vi "LTVDiffDriveCtrl_Pack_Ctrl_Params.vi"(4 "Max right vel ctrl effort V":dbl=12.0, 6 "Max left vel ctrl effort V":dbl=12.0, 7 "Desired X Pos Ctrl Tol M":dbl=0.0625, 8 "Desired Right Vel Ctrl Tol M/S":dbl=0.3, 9 "Desired Left Vel Ctrl Tol M/S":dbl=0.3, 10 "Desired Heading Ctrl Tol Rad":dbl=0.2, 11 "Desired Y Pos Meas Tol M":dbl=0.125) -> (3 "LTV_DiffDriveCtrl_Control":T1={"Max left vel ctrl effort V"=0.0, "Desired Heading Ctrl Tol Rad"=0.0, "Desired Y Pos Meas Tol M"=0.0, "Desired X Pos Ctrl Tol M"=0.2, "Desired Left Vel Ctrl Tol M/S"=0.2, "Desired Right Vel Ctrl Tol M/S"=0.1, "Max right vel ctrl effort V"=12.0} {"Max right vel ctrl effort V" format="%#_13g"; "Desired Right Vel Ctrl Tol M/S" format="%#_13g"; "Desired Left Vel Ctrl Tol M/S" format="%#_13g"; "Desired X Pos Ctrl Tol M" format="%#_13g"; "Desired Y Pos Meas Tol M" format="%#_13g"; "Desired Heading Ctrl Tol Rad" format="%#_13g"; "Max left vel ctrl effort V" format="%#_13g"})   [LabVIEW 2019, in "Trajectory_Library.lvlib"]
doc: "Pack control values for LTV Diff Drive Ctrl execute function\n\nInputs:\n - Desired X Pos Ctrl Tol -- double --- Maximum desired X position control tolerance (meters, Default: 0.0625)\n - Desired Y Pos Ctrl Tol -- double --- Maximum desired y position control tolerance (meters, Default: 0.125)\n - Desired Heading Ctrl Tol -- double --- Maximum desired heading control tolerance (meters, Default: 0.2)\n - Desired Left Vel Ctrl Tol -- double --- Maximum desired left velocity control tolerance (meters, Default: 0.3)\n - Desired Right Vel Ctrl Tol -- double --- Maximum desired right velocity control tolerance (meters, Default: 0.3)\n - Max left vel ctrl effort V -- double -- Maximum left motor dmd control effort (volts, default 12.0)\n - Max right vel ctrl effort V -- double -- Maximum right motor dmd control effort (volts, default 12.0)\n\nOutputs:\n - LTV Diff Drive Ctrl Control -- cluster -- Packed valules"
uses:
  Trajectory_Library.lvlib
  TypeDef/LTV_DIFF_DRIVE_CTRL_CONTROL_PARAMS.CTL
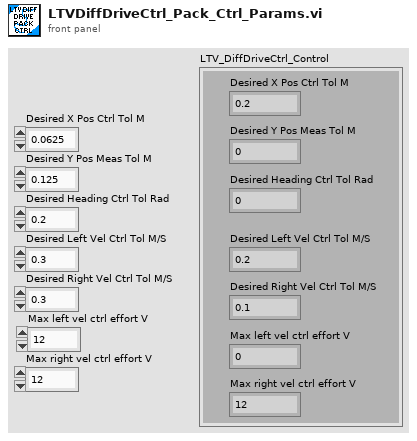
[diagram p1: front panel]
types:
  T1 = typedef "Trajectory_Library.lvlib/LTV_DIFF_DRIVE_CTRL_CONTROL_PARAMS.CTL" = cluster{"Max left vel ctrl effort V":dbl, "Desired Heading Ctrl Tol Rad":dbl, "Desired Y Pos Meas Tol M":dbl, "Desired X Pos Ctrl Tol M":dbl, "Desired Left Vel Ctrl Tol M/S":dbl, "Desired Right Vel Ctrl Tol M/S":dbl, "Max right vel ctrl effort V":dbl}
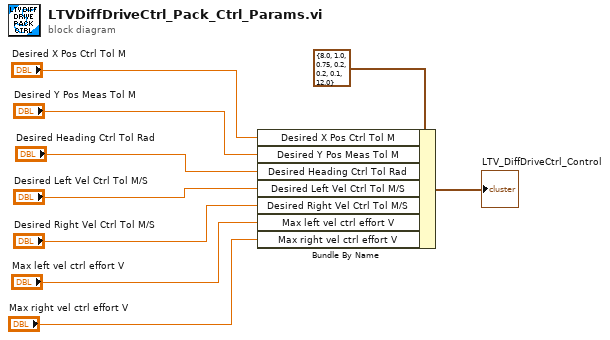
[diagram p0: block diagram]
diagram:
  n1 = Bundle By Name(cluster=T1 {"Max left vel ctrl effort V"=8.0, "Desired Heading Ctrl Tol Rad"=1.0, "Desired Y Pos Meas Tol M"=0.75, "Desired X Pos Ctrl Tol M"=0.2, "Desired Left Vel Ctrl Tol M/S"=0.2, "Desired Right Vel Ctrl Tol M/S"=0.1, "Max right vel ctrl effort V"=12.0} ("SngJntArmSim_Simulation _Params"), "Desired X Pos Ctrl Tol M"="Desired X Pos Ctrl Tol M", "Desired Y Pos Meas Tol M"="Desired Y Pos Meas Tol M", "Desired Heading Ctrl Tol Rad"="Desired Heading Ctrl Tol Rad", "Desired Left Vel Ctrl Tol M/S"="Desired Left Vel Ctrl Tol M/S", "Desired Right Vel Ctrl Tol M/S"="Desired Right Vel Ctrl Tol M/S", "Max left vel ctrl effort V"="Max left vel ctrl effort V", "Max right vel ctrl effort V"="Max right vel ctrl effort V") -> (→"LTV_DiffDriveCtrl_Control":T1)
